vi "PUBLIC.destructor.vi"(0 "i ref in":refnum<vi>, 5 "error in(no error)":errorcluster) -> (19 "error out":errorcluster)   [LabVIEW 2014]
doc: "This is the destructor of a class.\n\nLicense Agreement for this software:\n\nCopyright (C)\nGesellschaft für Schwerionenforschung, GSI\nPlanckstr. 1\n64291 Darmstadt\nGermany\n\nContact: D.Beck@gsi.de \n\nThis program is free software; you can redistribute it and/or modify it under the terms of the \nGNU General Public License as published by the Free Software Foundation; either version 2 of \nthe license, or (at your option) any later version.\n\nThis program is distributed in the hope that it will be useful, but WITHOUT ANY WARRANTY; \nwithout even the implied warranty of MERCHANTABILITY or FITNESS FOR A PARTICULAR PURPOSE. See the GNU General License for more details (http://www.gnu.org).\n\nGesellschaft für Schwerionenforschung, GSI\nPlanckstr. 1, 64291 Darmstadt, Germany\nFor all questions and ideas contact: M.Richter@gsi.de, H.Brand@gsi.de or D.Beck@gsi.de.\nLast update: 16-JUN-2004"
uses:
  UT_EField_DAQ_AnalogIO.lvlib
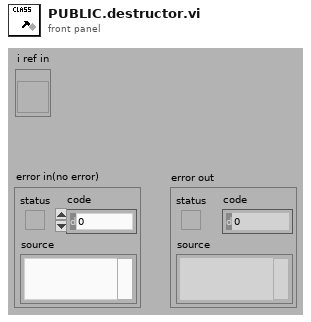
[diagram p1: front panel]
types:
  T1 = enum16{"SetAttribute", "GetAttribute", "CreateAttribute", "DestroyAttribute", "DestroyAllAtributes"}
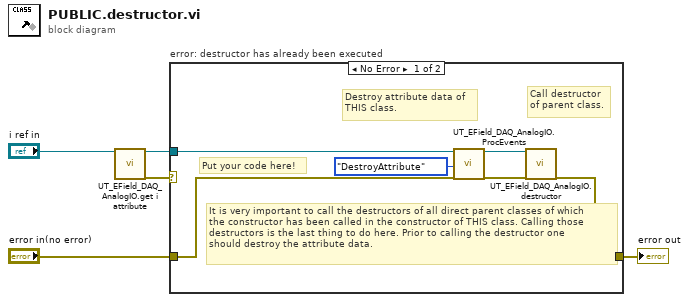
[diagram p0: block diagram]
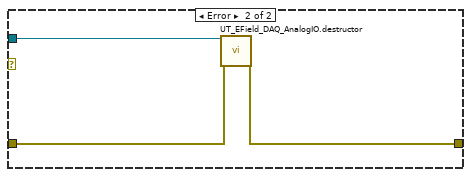
[diagram p2: hidden frame]
diagram:
  n1 = call "UT_EField_DAQ_AnalogIO.get i attribute.vi"("i ref in"="i ref in") -> ("i ref out"=w1:refnum<vi>, "error out"=w2:errorcluster)  [unwired: 16 in, 1 out]
  n2 = case "error: destructor has already been executed" shown="No Error" w2 {
    tunnel: [w8 w12] -> w5
    tunnel: "error in(no error)" -> [w7 w13]
    tunnel: w1 -> [w6 w14]
    frame No Error {
      # "It is very important to call the destructors of all direct parent classes of which\nthe constructor has been called in the constructor of THIS class. Calling those\ndestructors is the last thing to do here. Prior to calling the destructor one \nshould destroy the attribute data."
      # "Put your code here!"
      # "Destroy attribute data of \nTHIS class."
      # "Call destructor\nof parent class."
      n3 = call "UT_EField_DAQ_AnalogIO.ProcEvents.vi"("i ref in"=w6, 3:T1."DestroyAttribute" ("Action"), "error in"=w7) -> ("i ref out"=w10:refnum<vi>, "error out"=w9:errorcluster)  [unwired: 15 in]
      n4 = call "UT_EField_DAQ_AnalogIO.destructor.vi"("i ref in"=w10, "error in(no error)"=w9) -> ("error out"=w8:errorcluster)  [unwired: 17 in]
    }
    frame Error {
      n5 = call "UT_EField_DAQ_AnalogIO.destructor.vi"("i ref in"=w14, "error in(no error)"=w13) -> ("error out"=w12:errorcluster)  [unwired: 17 in]
    }
  }
  "error out" <- w5
